vi "Simpler FPGA tester.vi"(4 "error in":errorcluster, 6 "Repetitions":dbl=1.0, 7 "Photon number":u16) -> (0 "error IO":errorcluster, 3 "Time":dbl)   [LabVIEW 2013]
uses:
  <vilib>/DAQmx/write.llb/DAQmx Write (Digital Bool 1Line 1Point).vi
  <vilib>/DAQmx/read.llb/DAQmx Read (Digital Bool 1Line 1Point).vi
  <vilib>/DAQmx/read.llb/DAQmx Read (Counter DBL 1Chan 1Samp).vi
  <vilib>/DAQmx/create/channels.llb/DAQmx Create Channel (CI-Pulse Width).vi
  <vilib>/DAQmx/miscellaneous.llb/DAQmx Fill In Error Info.vi
  <resource>/objmgr/daqmx.rc
panel:
  in  "Delay":u32
  in  "GPIB address":string="15"
  out "Set 1":bool[](array[boolean])
  out "Set 2":bool[](array[boolean])
  out "Set 3":bool[](array[boolean])
  out "Set 4":bool[](array[boolean])
  out "16-bit number":bool[](array[boolean])
  # "Or specify levels below:"
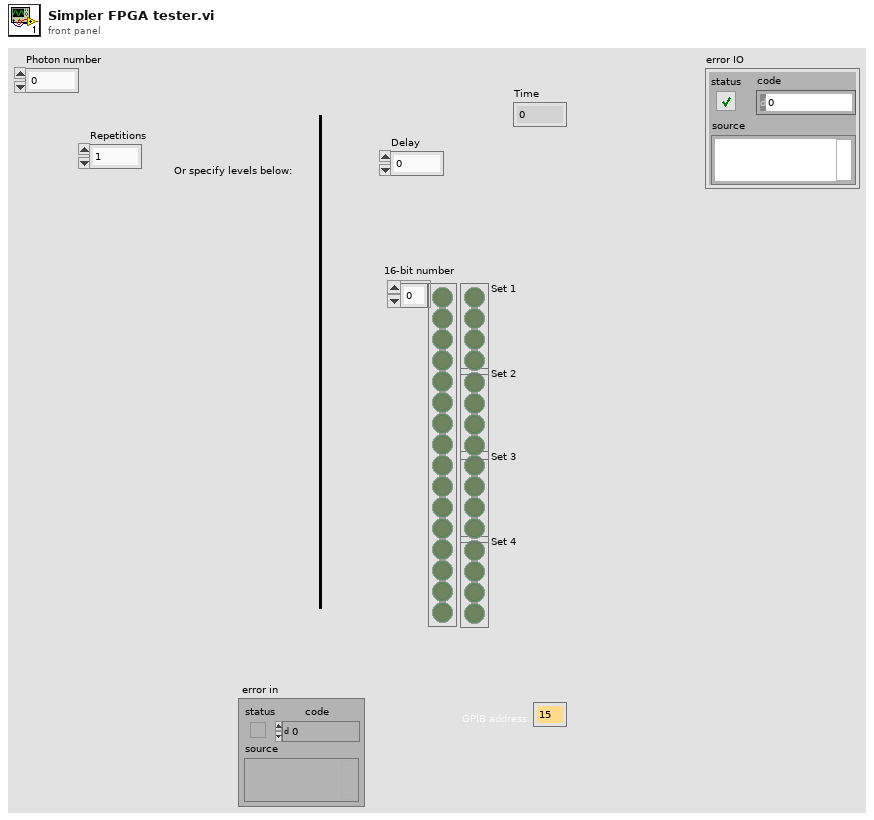
[diagram p1: front panel]
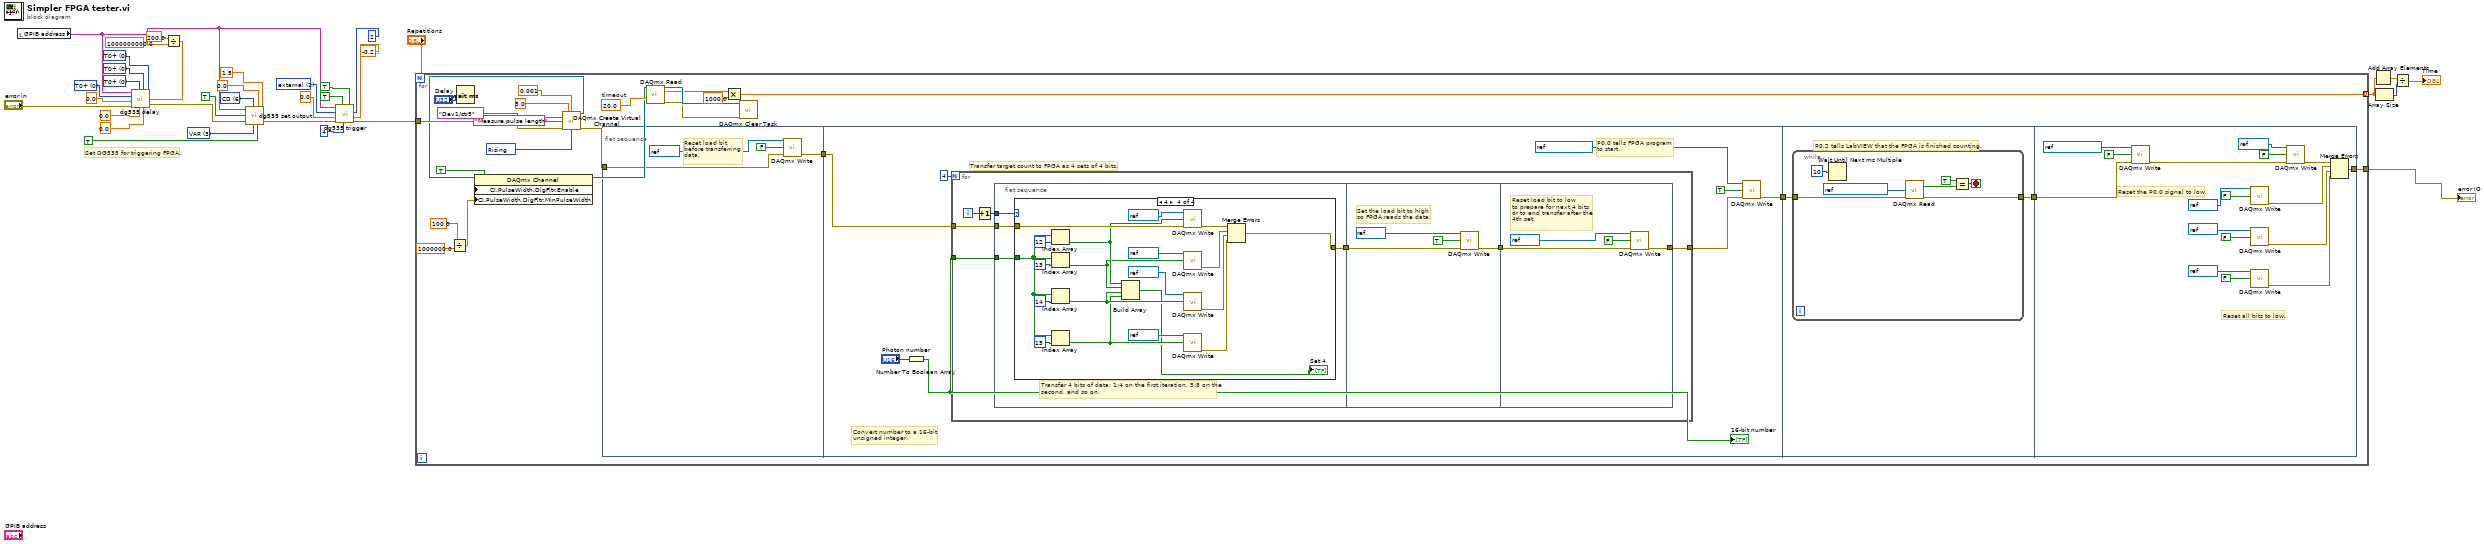
[diagram p0: block diagram]
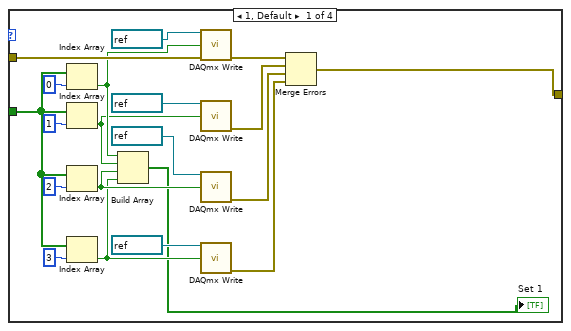
[diagram p2: hidden frame]
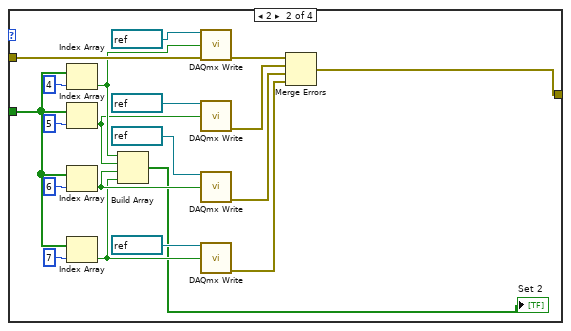
[diagram p3: hidden frame]
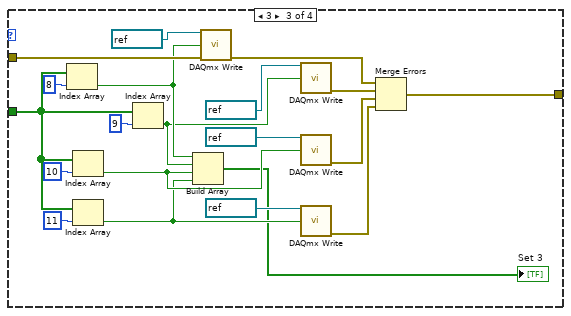
[diagram p4: hidden frame]
diagram:
  w23 = u32 1 items=["internal", "external", "single shot", "burst", "line"] ("trigger")
  w25 = 3 items=["TTL", "NIM", "ECL", "VAR"] ("mode")
  w27 = u16 6 items=["T0", "A", "B", "AB", "C", "D", "CD"] ("output")
  w30 = u32 0 items=["T0+", "A+", "B+", "C+"] ("D=")
  w31 = u32 0 items=["T0+", "A+", "B+", "D+"] ("C=")
  w32 = u32 0 items=["T0+", "A+", "C+", "D+"] ("B=")
  w33 = u32 0 items=["T0+", "B+", "C+", "D+"] ("A=")
  # "Set DG535 for triggering FPGA."
  n1 = local read "GPIB address"() -> (w15:string)
  n2 = Divide(x=200.0 ("D"), y=1000000000.0) -> (x/y=w9:dbl)
  n3 = call "dg535 delay.vi"("C"=0.0, "D"=w9, "D="=w30, "C="=w31, "B"=0.0 ("C"), "error in"="error in", "A"=0.0 ("D"), "B="=w32, "A="=w33, "GPIB address"=w15) -> ("error out"=w29:errorcluster)
  n4 = call "dg535 set output.vi"("GPIB address"=w15, "output"=w27, "set"=TRUE, "error in"=w29, "mode"=w25, "offset"=0.0, "amplitude"=1.5, "load"=TRUE) -> ("error out"=w16:errorcluster)  [unwired: 1 in]
  n5 = call "dg535 trigger.vi"("external trigger level"=sgl -0.2, "burst count"=2, "trigger slope"=TRUE, "burst period"=4, "input impedance"=TRUE, "error in"=w16, "internal/burst trigger rate"=0.0, "trigger"=w23, "GPIB address"=w15) -> ("error out"=w8:errorcluster)
  n6 = for {
    N: "Repetitions" -> [_]
    tunnel: [w45] -> w2 mode=indexing
    tunnel: w8 -> [w44]
    tunnel: [w42] -> w1
    w49 = 20.0  # timeout
    w52 = 10280 items=["Rising"=10280, "Falling"=10171] ("Starting Edge")
    n7 = Divide(x=100.0 ("CI.PulseWidth.DigFltr.MinPulseWidth"), y=1000000.0) -> (x/y=w35:dbl)
    n8 = Wait (ms)(milliseconds to wait="Delay") -> ()  [unwired: 1 out]
    n9 = call-poly <vilib>:"DAQmx Create Virtual Channel.vi"("maximum value"=5.0 ("Maximum Value (sec)"), "minimum value"=0.001 ("Minimum Value (sec)"), "counter"=tag "Dev1/ctr3" ("Physical Channel"), "name to assign"="Measure pulse length", "error in"=w44, "starting edge"=w52) -> ("task out"=w40:refnum<k21>, "error out"=w46:errorcluster)  [unwired: 8 in]
    n10 = property class="DAQmx Channel"(reference=w40, "CI.PulseWidth.DigFltr.Enable"=TRUE, "CI.PulseWidth.DigFltr.MinPulseWidth"=w35) -> (reference out=w39:refnum<k21>)  [unwired: 1 in, 1 out]
    n11 = flat-sequence {
      tunnel: w46 -> [w60]
      tunnel: [w59] -> w58
      tunnel: [w65] -> w57
      tunnel: w58 -> [w69]
      tunnel: w57 -> [w171]
      tunnel: [w170] -> w56
      tunnel: [w179] -> w42
      tunnel: w56 -> [w185]
      frame #0 {
        # "Reset load bit\nbefore transferring\ndata."
        n12 = call-poly <vilib>:"DAQmx Write.vi"("task/channels in"=refnum<k21> "BIT5", "data"=FALSE, "error in"=w60) -> ("error out"=w59:errorcluster)  [unwired: 10 in, 2 out]
      }
      frame #1 {
        # "P0.0 tells FPGA program \nto start."
        # "Convert number to a 16-bit\nunsigned integer."
        # "Transfer target count to FPGA as 4 sets of 4 bits."
        n13 = Number To Boolean Array(number="Photon number") -> (Boolean array=w64:bool[])
        "16-bit number" <- w64
        n14 = for {
          N: 4 -> [_]
          tunnel: w64 -> [w74]
          tunnel: w69 -> [w76]
          tunnel: [w71] -> w66
          i -> [w77]
          n15 = Increment(x=w77) -> (x+1=w75:i32)
          n16 = flat-sequence {
            tunnel: w76 -> [w81]
            tunnel: w75 -> [w80]
            tunnel: w74 -> [w79]
            tunnel: [w78] -> w73
            tunnel: w73 -> [w163]
            tunnel: [w162] -> w72
            tunnel: w72 -> [w167]
            tunnel: [w166] -> w71
            frame #0 {
              # "Transfer 4 bits of data: 1:4 on the first iteration, 5:8 on the\nsecond, and so on."
              n17 = case shown="4" w80 {
                tunnel: w79 -> [w89 w109 w129 w149]
                tunnel: w81 -> [w88 w108 w128 w148]
                tunnel: [w87 w107 w127 w147] -> w78
                frame 1, Default {
                  n18 = Index Array(array=w89, index=0) -> (element=w86:bool)
                  n19 = Index Array(array=w89, index=1) -> (element=w85:bool)
                  n20 = Index Array(array=w89, index=2) -> (element=w84:bool)
                  n21 = Index Array(array=w89, index=3) -> (element=w83:bool)
                  n22 = Build Array(w86, w85, w84, w83) -> (→"Set 1":bool[])
                  n23 = call-poly <vilib>:"DAQmx Write.vi"("task/channels in"=refnum<k21> "BIT1", "data"=w86, "error in"=w88) -> ("error out"=w97:errorcluster)  [unwired: 10 in, 2 out]
                  n24 = call-poly <vilib>:"DAQmx Write.vi"("task/channels in"=refnum<k21> "BIT2", "data"=w85) -> ("error out"=w96:errorcluster)  [unwired: 11 in, 2 out]
                  n25 = call-poly <vilib>:"DAQmx Write.vi"("task/channels in"=refnum<k21> "BIT3", "data"=w84) -> ("error out"=w95:errorcluster)  [unwired: 11 in, 2 out]
                  n26 = call-poly <vilib>:"DAQmx Write.vi"("task/channels in"=refnum<k21> "BIT4", "data"=w83) -> ("error out"=w94:errorcluster)  [unwired: 11 in, 2 out]
                  n27 = Merge Errors(w97, w96, w95, w94) -> (w87:errorcluster)
                }
                frame 2 {
                  n28 = Index Array(array=w109, index=4) -> (element=w106:bool)
                  n29 = Index Array(array=w109, index=5) -> (element=w105:bool)
                  n30 = Index Array(array=w109, index=6) -> (element=w104:bool)
                  n31 = Index Array(array=w109, index=7) -> (element=w103:bool)
                  n32 = Build Array(w106, w105, w104, w103) -> (→"Set 2":bool[])
                  n33 = call-poly <vilib>:"DAQmx Write.vi"("task/channels in"=refnum<k21> "BIT1", "data"=w106, "error in"=w108) -> ("error out"=w117:errorcluster)  [unwired: 10 in, 2 out]
                  n34 = call-poly <vilib>:"DAQmx Write.vi"("task/channels in"=refnum<k21> "BIT2", "data"=w105) -> ("error out"=w116:errorcluster)  [unwired: 11 in, 2 out]
                  n35 = call-poly <vilib>:"DAQmx Write.vi"("task/channels in"=refnum<k21> "BIT3", "data"=w104) -> ("error out"=w115:errorcluster)  [unwired: 11 in, 2 out]
                  n36 = call-poly <vilib>:"DAQmx Write.vi"("task/channels in"=refnum<k21> "BIT4", "data"=w103) -> ("error out"=w114:errorcluster)  [unwired: 11 in, 2 out]
                  n37 = Merge Errors(w117, w116, w115, w114) -> (w107:errorcluster)
                }
                frame 3 {
                  n38 = Index Array(array=w129, index=8) -> (element=w126:bool)
                  n39 = Index Array(array=w129, index=10) -> (element=w124:bool)
                  n40 = Index Array(array=w129, index=11) -> (element=w123:bool)
                  n41 = Index Array(array=w129, index=9) -> (element=w125:bool)
                  n42 = Build Array(w126, w125, w124, w123) -> (→"Set 3":bool[])
                  n43 = call-poly <vilib>:"DAQmx Write.vi"("task/channels in"=refnum<k21> "BIT1", "data"=w126, "error in"=w128) -> ("error out"=w137:errorcluster)  [unwired: 10 in, 2 out]
                  n44 = call-poly <vilib>:"DAQmx Write.vi"("task/channels in"=refnum<k21> "BIT2", "data"=w125) -> ("error out"=w136:errorcluster)  [unwired: 11 in, 2 out]
                  n45 = call-poly <vilib>:"DAQmx Write.vi"("task/channels in"=refnum<k21> "BIT3", "data"=w124) -> ("error out"=w135:errorcluster)  [unwired: 11 in, 2 out]
                  n46 = call-poly <vilib>:"DAQmx Write.vi"("task/channels in"=refnum<k21> "BIT4", "data"=w123) -> ("error out"=w134:errorcluster)  [unwired: 11 in, 2 out]
                  n47 = Merge Errors(w137, w136, w135, w134) -> (w127:errorcluster)
                }
                frame 4 {
                  n48 = Index Array(array=w149, index=12) -> (element=w146:bool)
                  n49 = Index Array(array=w149, index=13) -> (element=w145:bool)
                  n50 = Index Array(array=w149, index=14) -> (element=w144:bool)
                  n51 = Index Array(array=w149, index=15) -> (element=w143:bool)
                  n52 = Build Array(w146, w145, w144, w143) -> (→"Set 4":bool[])
                  n53 = call-poly <vilib>:"DAQmx Write.vi"("task/channels in"=refnum<k21> "BIT1", "data"=w146, "error in"=w148) -> ("error out"=w157:errorcluster)  [unwired: 10 in, 2 out]
                  n54 = call-poly <vilib>:"DAQmx Write.vi"("task/channels in"=refnum<k21> "BIT2", "data"=w145) -> ("error out"=w156:errorcluster)  [unwired: 11 in, 2 out]
                  n55 = call-poly <vilib>:"DAQmx Write.vi"("task/channels in"=refnum<k21> "BIT3", "data"=w144) -> ("error out"=w155:errorcluster)  [unwired: 11 in, 2 out]
                  n56 = call-poly <vilib>:"DAQmx Write.vi"("task/channels in"=refnum<k21> "BIT4", "data"=w143) -> ("error out"=w154:errorcluster)  [unwired: 11 in, 2 out]
                  n57 = Merge Errors(w157, w156, w155, w154) -> (w147:errorcluster)
                }
              }
            }
            frame #1 {
              # "Set the load bit to high\nso FPGA reads the data."
              n58 = call-poly <vilib>:"DAQmx Write.vi"("task/channels in"=refnum<k21> "BIT5", "data"=TRUE, "error in"=w163) -> ("error out"=w162:errorcluster)  [unwired: 10 in, 2 out]
            }
            frame #2 {
              # "Reset load bit to low\nto prepare for next 4 bits\nor to end transfer after the\n4th set."
              n59 = call-poly <vilib>:"DAQmx Write.vi"("task/channels in"=refnum<k21> "BIT5", "data"=FALSE, "error in"=w167) -> ("error out"=w166:errorcluster)  [unwired: 10 in, 2 out]
            }
          }
        }
        n60 = call-poly <vilib>:"DAQmx Write.vi"("task/channels in"=refnum<k21> "LaserChannel", "data"=TRUE, "error in"=w66) -> ("error out"=w65:errorcluster)  [unwired: 10 in, 2 out]
      }
      frame #2 {
        # "P0.2 tells LabVIEW that the FPGA is finished counting."
        n61 = while {
          tunnel: w171 -> [w178]
          tunnel: [w177] -> w170
          stop <- w174 stop-if-true
          n62 = Wait Until Next ms Multiple(millisecond multiple=u32 10) -> ()  [unwired: 1 out]
          n63 = call-poly <vilib>:"DAQmx Read.vi"("task/channels in"=refnum<k21> "P02countSignal", "error in"=w178) -> ("data"=w175:bool, "error out"=w177:errorcluster)  [unwired: 11 in, 1 out]
          n64 = Equal?(x=TRUE, y=w175) -> (x = y?=w174:bool)
        }
      }
      frame #3 {
        # "Reset all bits to low."
        # "Reset the P0.0 signal to low."
        n65 = call-poly <vilib>:"DAQmx Write.vi"("task/channels in"=refnum<k21> "LaserChannel", "data"=FALSE, "error in"=w185) -> ("error out"=w184:errorcluster)  [unwired: 10 in, 2 out]
        n66 = call-poly <vilib>:"DAQmx Write.vi"("task/channels in"=refnum<k21> "BIT2", "data"=FALSE) -> ("error out"=w192:errorcluster)  [unwired: 11 in, 2 out]
        n67 = call-poly <vilib>:"DAQmx Write.vi"("task/channels in"=refnum<k21> "BIT3", "data"=FALSE) -> ("error out"=w191:errorcluster)  [unwired: 11 in, 2 out]
        n68 = call-poly <vilib>:"DAQmx Write.vi"("task/channels in"=refnum<k21> "BIT4", "data"=FALSE) -> ("error out"=w190:errorcluster)  [unwired: 11 in, 2 out]
        n69 = call-poly <vilib>:"DAQmx Write.vi"("task/channels in"=refnum<k21> "BIT1", "data"=FALSE, "error in"=w184) -> ("error out"=w193:errorcluster)  [unwired: 10 in, 2 out]
        n70 = Merge Errors(w193, w192, w191, w190) -> (w179:errorcluster)
      }
    }
    n71 = call-poly <vilib>:"DAQmx Read.vi"("task/channels in"=w39, "timeout"=w49) -> ("task out"=w51:refnum<k21>, "data"=w47:dbl, "error out"=w50:errorcluster)  [unwired: 11 in]
    n72 = Multiply(x=w47, y=1000.0) -> (x*y=w45:dbl)
    n73 = call <vilib>:"DAQmx Clear Task.vi"("task in"=w51, "error in"=w50) -> ()  [unwired: 13 in, 1 out]
  }
  "error IO" <- w1
  n74 = Add Array Elements(numeric array=w2) -> (sum=w4:dbl)
  n75 = Array Size(array=w2) -> (size(s)=w3:i32)
  n76 = Divide(x=w4, y=w3) -> (x/y=→"Time":dbl)
